vi "Read Timing Source Properties.vi"(8 "error in (no error)":errorcluster, 11 "CustomDeviceRepo in":refnum<class "CustomDeviceRepo.lvclass">) -> (0 "error out":errorcluster, 2 "Timing Source Properties":T1, 3 "CustomDeviceRepo out":refnum<class "CustomDeviceRepo.lvclass">)   [LabVIEW 2019, in "CustomDeviceRepo.lvclass"]
uses:
  CustomDeviceRepo.lvclass
  XML Controls/Timing Source Properties.ctl
  XML Controls/Timing Source Source Distribution Properties.ctl
  XML Controls/Supported Targets.ctl
  XML Controls/Path Cluster.ctl
  CustomDeviceRepo.lvclass/CustomDeviceRepo.ctl
  VeriStand Custom Device XML Parser.lvlib
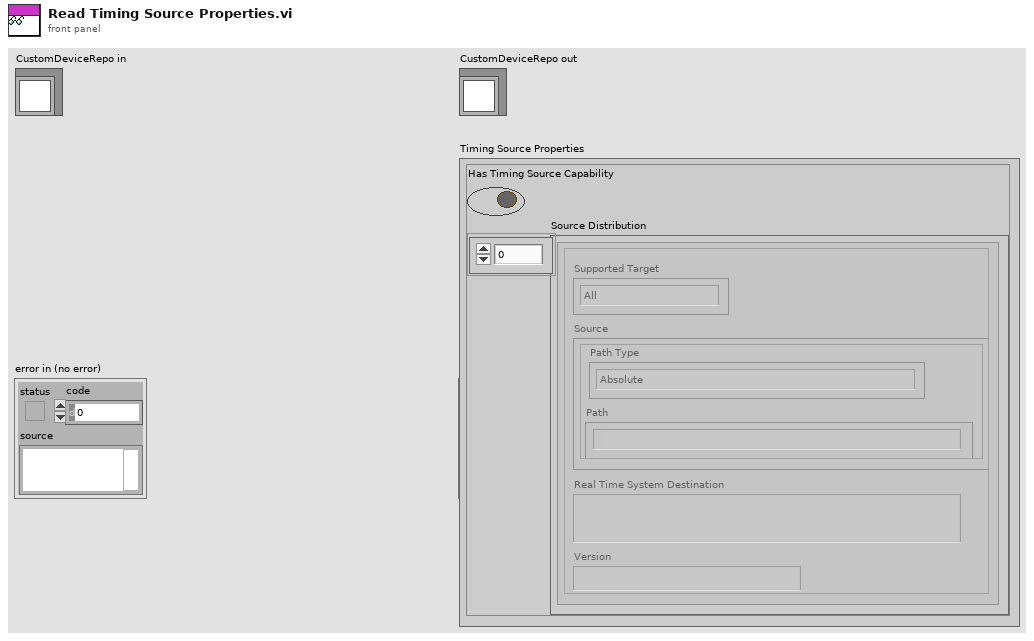
[diagram p1: front panel]
types:
  T1 = typedef "VeriStand Custom Device XML Parser.lvlib/Timing Source Properties.ctl" = cluster{"Has Timing Source Capability":bool, "Source Distribution":T2}
  T2 = typedef "VeriStand Custom Device XML Parser.lvlib/Timing Source Source Distribution Properties.ctl" = cluster{"Supported Target":T3, "Source":T4, "Real Time System Destination":string, "Version":string}[]
  T3 = typedef "VeriStand Custom Device XML Parser.lvlib/Supported Targets.ctl" = enum16{"All", "Pharlap", "VxWorks", "Windows", "Linux_32_ARM", "Linux_x64", "PharlapWindows", "PharlapVxWorks", "VxWorksWindows"}
  T4 = typedef "VeriStand Custom Device XML Parser.lvlib/Path Cluster.ctl" = cluster{"Path":path, "Path Type":enum16{"Absolute", "To Base", "To Common Doc Dir", "To Application Data Dir"}}
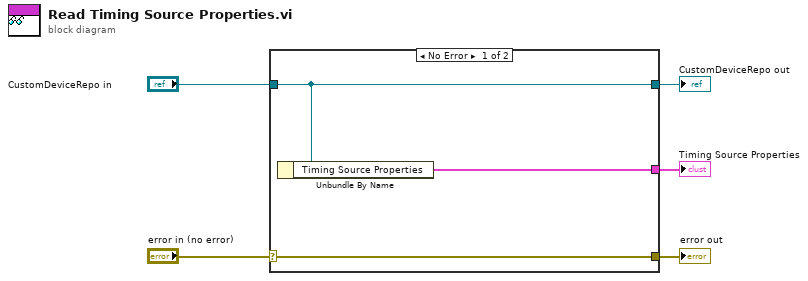
[diagram p0: block diagram]
diagram:
  n1 = case shown="No Error" "error in (no error)" {
    selector: "error in (no error)" -> [w8 w9]
    tunnel: [w8 w9] -> w4
    tunnel: [w7 w10] -> w2
    tunnel: "CustomDeviceRepo in" -> [w7 w10]
    tunnel: [w6 _] -> w1
    frame No Error {
      n2 = Unbundle By Name(w7) -> ("Timing Source Properties"=w6:T1)
    }
    frame Error {
    }
  }
  "error out" <- w4
  "CustomDeviceRepo out" <- w2
  "Timing Source Properties" <- w1
